vi "Keithley 2400 IV sweep.vi"(0 "VISA resource name":refnum<visa-resource-name>, 1 "Filter Count (1)":i32=1, 2 "Settling (ms)":u32=500, 3 "Current limit (0.1)":dbl=0.1, 9 "Voltage points":dbl[](array[numeric]), 11 "error in (no error)":errorcluster, 12 "Stop occurrence":refnum<k4>, 13 "XY Graph to update":refnum<vi>, 14 "Status String Reference":refnum<vi>) -> (4 "VISA resource name out":refnum<visa-resource-name>, 6 "Current points":dbl[](array[numeric]), 8 "Voltage points (Collected)":dbl[](array[numeric]), 15 "error out":errorcluster)   [LabVIEW 2019]
uses:
  <instrlib>/Keithley 2450/Keithley 2450.lvlib
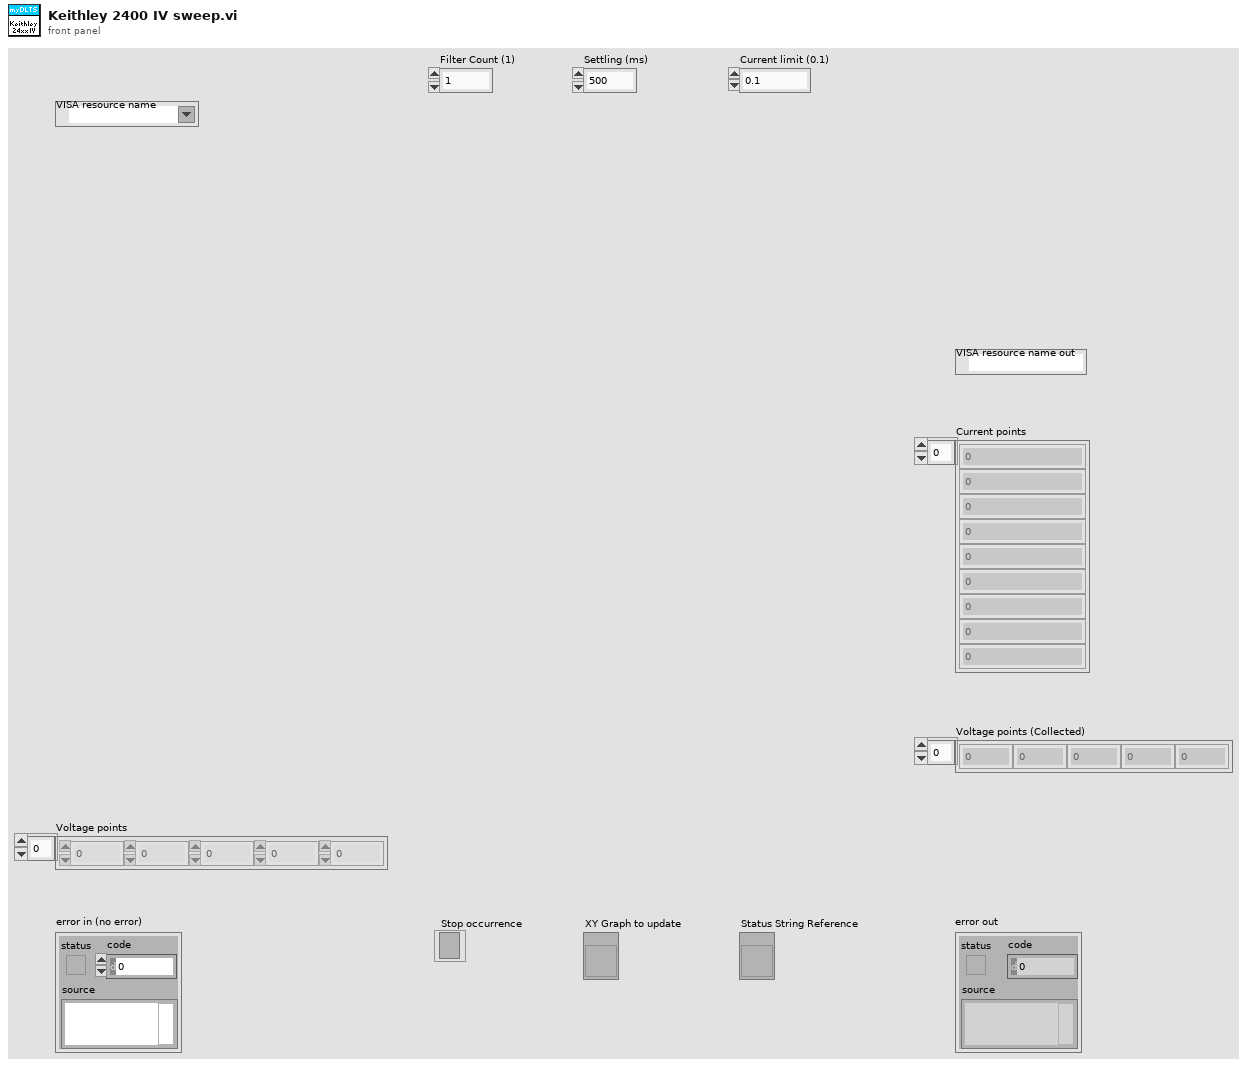
[diagram p1: front panel]
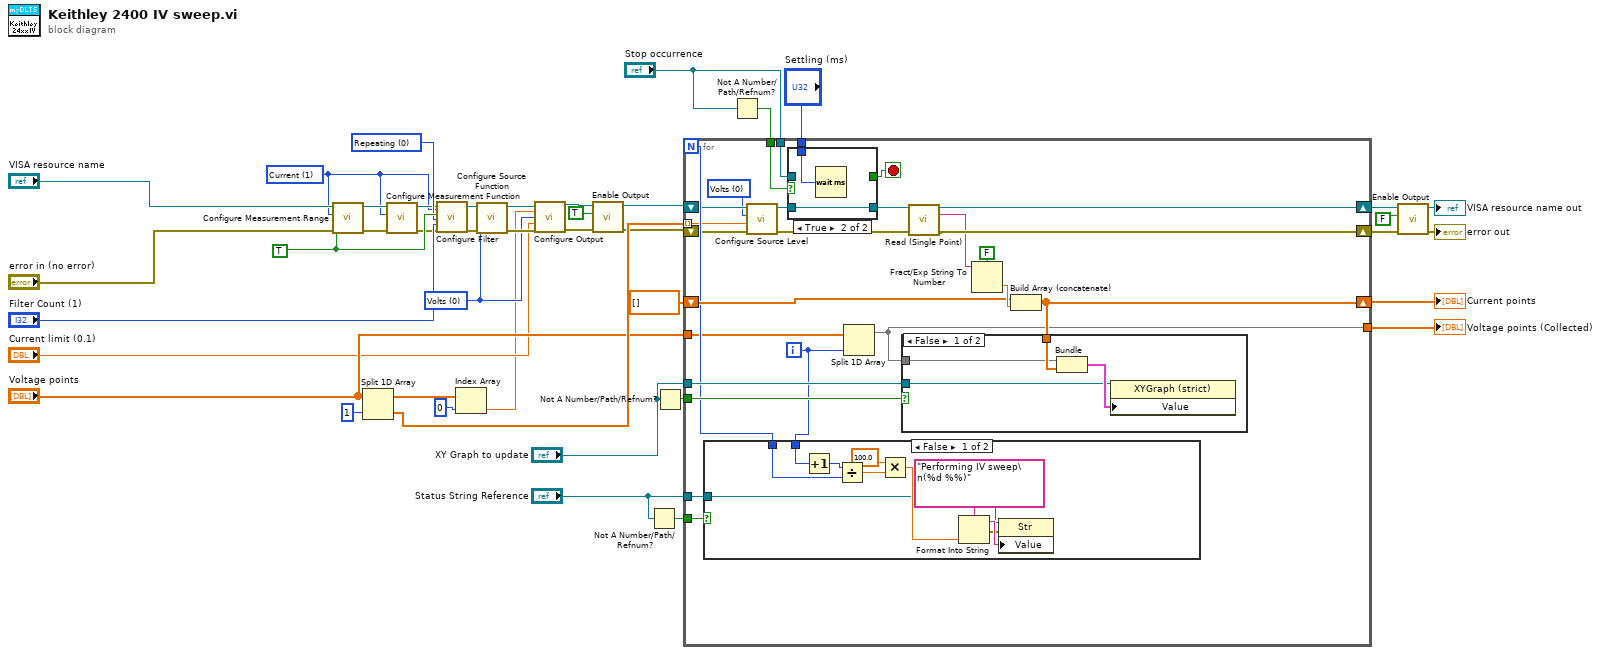
[diagram p0: block diagram]
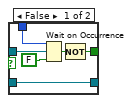
[diagram p2: hidden frame]
diagram:
  w18 = u16 0 items=["Volts", "Current"] ("Function (0: Volts)")
  w24 = u16 0 items=["Repeating", "Moving"] ("Filter Type  (0: Repeating)")
  w11 = u16 1 items=["Volts", "Current", "Resistance"] ("Function (0: Volts)")
  w25 = TRUE ("Enable Auto Range (T:Enable)")
  n1 = call <instrlib>:"Configure Measurement Range.vi"("error in (no error)"="error in (no error)", "Enable Auto Range (T:Enable)"=w25, "Function (0: Volts)"=w11, "VISA resource name"="VISA resource name") -> ("error out"=w14:errorcluster, "VISA resource name out"=w15:refnum<visa-resource-name>)  [unwired: 6 in]
  n2 = Split 1D Array(array="Voltage points", index=1) -> (first subarray=w41:dbl[], second subarray=w37:dbl[])
  n3 = call <instrlib>:"Configure Measurement Function.vi"("error in (no error)"=w14, "Function (0: Volts)"=w11, "VISA resource name"=w15) -> ("error out"=w12:errorcluster, "VISA resource name out"=w13:refnum<visa-resource-name>)  [unwired: 7 in]
  n4 = call <instrlib>:"Configure Filter.vi"("VISA resource name"=w13, "Function (0: Volts)"=w11, "Enable Filter  (T: Enable)"=w25, "Filter Type  (0: Repeating)"=w24, "Number of Filter Readings (3)"="Filter Count (1)", "error in (no error)"=w12) -> ("VISA resource name out"=w22:refnum<visa-resource-name>, "error out"=w21:errorcluster)  [unwired: 12 in]
  n5 = Index Array(array=w41, index=0) -> (element=w16:dbl)
  n6 = call <instrlib>:"Configure Source Function.vi"("error in (no error)"=w21, "Function (0: Volts)"=w18, "VISA resource name"=w22) -> ("error out"=w19:errorcluster, "VISA resource name out"=w20:refnum<visa-resource-name>)  [unwired: 7 in]
  n7 = call <instrlib>:"Configure Output.vi"("VISA resource name"=w20, "Source Level (0)"=w16, "Source Mode  (0: Voltage)"=w18, "Source Limit Level (0.1)"="Current limit (0.1)", "error in (no error)"=w19) -> ("VISA resource name out"=w9:refnum<visa-resource-name>, "error out"=w10:errorcluster)  [unwired: 9 in]
  n8 = call <instrlib>:"Enable Output.vi"("error in (no error)"=w10, "Enable Output (T: Enable)"=TRUE, "VISA resource name"=w9) -> ("error out"=w6:errorcluster, "VISA resource name out"=w7:refnum<visa-resource-name>)  [unwired: 7 in]
  n9 = Not A Number/Path/Refnum?(number/path/refnum="Status String Reference") -> (NaN/Path/Refnum?=w35:bool)
  n10 = Not A Number/Path/Refnum?(number/path/refnum="XY Graph to update") -> (NaN/Path/Refnum?=w36:bool)
  n11 = Not A Number/Path/Refnum?(number/path/refnum="Stop occurrence") -> (NaN/Path/Refnum?=w33:bool)
  n12 = for {
    N -> [w60]
    tunnel: w37 -> [w50] mode=indexing
    shift-right: [w44] -> w5
    shift-left: w6 -> [w51]
    shift-right: [w45] -> w4
    shift-left: w7 -> [w52]
    tunnel: "Settling (ms)" -> [w58]
    shift-right: [w65] -> w38
    shift-left: dbl[] [] -> [w66]
    tunnel: "Voltage points" -> [w54]
    tunnel: "XY Graph to update" -> [w64]
    tunnel: w36 -> [w63]
    tunnel: w35 -> [w62]
    tunnel: "Status String Reference" -> [w61]
    tunnel: w33 -> [w56]
    tunnel: "Stop occurrence" -> [w55]
    tunnel: [w53] -> w29
    i -> [w59]
    stop <- w57 stop-if-true
    w49 = u16 0 items=["Volts", "Current"] ("Function (0: Volts)")
    n13 = case shown="False" w62 {
      tunnel: w61 -> [w77 _]
      tunnel: w60 -> [w84 _]
      tunnel: w59 -> [w86 _]
      frame False {
        n14 = Increment(x=w86) -> (x+1=w85:i32)
        n15 = Divide(x=w85, y=w84) -> (x/y=w83:dbl)
        n16 = Multiply(x=100.0, y=w83) -> (x*y=w78:dbl)
        n17 = Format Into String(format string="Performing IV sweep\n(%d %%)", w78) -> (resulting string=w81:string, error out=w80:errorcluster)  [unwired: 2 in]
        n18 = property class="Str"(reference=w77, error in=w80, "Value"=w81) -> ()  [unwired: 2 out]
      }
      frame True {
      }
    }
    n19 = call <instrlib>:"Configure Source Level.vi"("error in (no error)"=w51, "Source Level (1.0)"=w50, "Function (0: Volts)"=w49, "VISA resource name"=w52) -> ("error out"=w46:errorcluster, "VISA resource name out"=w48:refnum<visa-resource-name>)  [unwired: 6 in]
    n20 = case shown="True" w56 {
      tunnel: [w73 _] -> w57
      tunnel: w58 -> [w72 w76]
      tunnel: w55 -> [w71 _]
      tunnel: w48 -> [w69 w75]
      tunnel: [w69 w75] -> w47
      frame False {
        n21 = Wait on Occurrence(1:FALSE ("ignore previous (T)"), 2:w71, 3:w72) -> (0:w74:bool)
        n22 = Not(x=w74) -> (.not. x?=w73:bool)
      }
      frame True {
        n23 = Wait (ms)(milliseconds to wait=w76) -> ()  [unwired: 1 out]
      }
    }
    n24 = Split 1D Array(array=w54, index=w59) -> (first subarray=w53:dbl[])  [unwired: 1 out]
    n25 = call <instrlib>:"Read (Single Point).vi"("VISA resource name"=w47, "error in (no error)"=w46) -> ("VISA resource name out"=w45:refnum<visa-resource-name>, "Data out"=w43:string, "error out"=w44:errorcluster)  [unwired: 11 in]
    n26 = Fract/Exp String To Number(use system decimal point (T)=FALSE, string=w43) -> (number=w67:dbl)  [unwired: 2 in, 1 out]
    n27 = Build Array (concatenate)(w66, w67) -> (w65:dbl[])
    n28 = case shown="False" w63 {
      tunnel: w65 -> [w90 _]
      tunnel: w64 -> [w88 _]
      tunnel: w53 -> [w87 _]
      frame False {
        n29 = Bundle(w87, w90) -> (w89:cluster{dbl[], dbl[]})  [unwired: 1 in]
        n30 = property on="Property Node" class="XYGraph (strict)"(reference=w88, "Value"=w89) -> ()  [unwired: 1 in, 2 out]
      }
      frame True {
      }
    }
  }
  "Current points" <- w38
  "Voltage points (Collected)" <- w29
  n31 = call <instrlib>:"Enable Output.vi"("error in (no error)"=w5, "Enable Output (T: Enable)"=FALSE ("Output (Off)"), "VISA resource name"=w4) -> ("error out"=→"error out":errorcluster, "VISA resource name out"=→"VISA resource name out":refnum<visa-resource-name>)  [unwired: 7 in]
